vi "Get Source Read Back State.vi"(8 "error in (no error)":errorcluster, 11 "VISA resource name":refnum<visa-resource-name>) -> (0 "error out":errorcluster, 1 "Current Read Back Enabled?":bool, 2 "Voltage Read Back Enabled?":bool, 3 "VISA resource name out":refnum<visa-resource-name>)   [LabVIEW 2020, in "Keithley 2450.lvlib"]
doc: "Gets state of Source Read Back on the instrument."
uses:
  Keithley 2450.lvlib
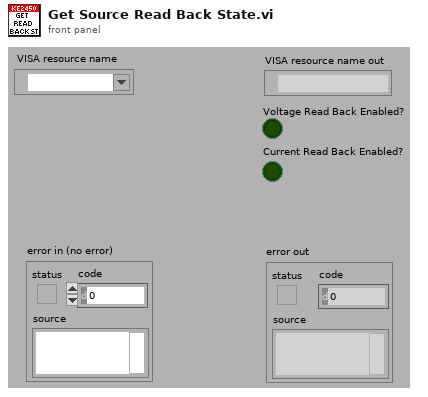
[diagram p1: front panel]
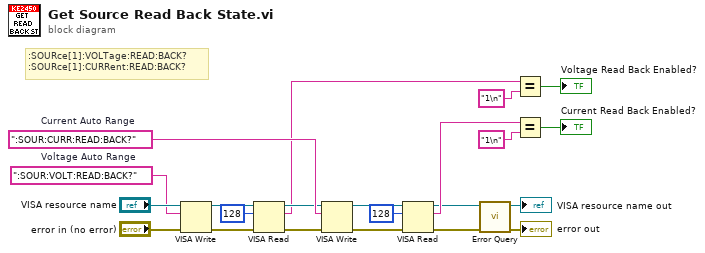
[diagram p0: block diagram]
diagram:
  w8 = ":SOUR:CURR:READ:BACK?"  # Current Auto Range
  w9 = ":SOUR:VOLT:READ:BACK?"  # Voltage Auto Range
  # ":SOURce[1]:VOLTage:READ:BACK?\n:SOURce[1]:CURRent:READ:BACK?"
  n1 = VISA Write(VISA resource name="VISA resource name", write buffer=w9, error in (no error)="error in (no error)") -> (VISA resource name out=w21:refnum<visa-resource-name>, error out=w22:errorcluster)  [unwired: 1 out]
  n2 = VISA Read(VISA resource name=w21, byte count=u32 128, error in (no error)=w22) -> (VISA resource name out=w7:refnum<visa-resource-name>, read buffer=w6:string, error out=w10:errorcluster)  [unwired: 1 out]
  n3 = VISA Write(VISA resource name=w7, write buffer=w8, error in (no error)=w10) -> (VISA resource name out=w13:refnum<visa-resource-name>, error out=w12:errorcluster)  [unwired: 1 out]
  n4 = VISA Read(VISA resource name=w13, byte count=u32 128, error in (no error)=w12) -> (VISA resource name out=w2:refnum<visa-resource-name>, read buffer=w5:string, error out=w1:errorcluster)  [unwired: 1 out]
  n5 = call "Error Query.vi"("error in (no error)"=w1, "VISA resource name"=w2) -> ("error out"=→"error out":errorcluster, "VISA resource name out"=→"VISA resource name out":refnum<visa-resource-name>)  [unwired: 8 out]
  n6 = Equal?(x=w6, y="1\n") -> (x = y?=→"Voltage Read Back Enabled?":bool)
  n7 = Equal?(x=w5, y="1\n") -> (x = y?=→"Current Read Back Enabled?":bool)
